vi "Get All Symbol Notifications.vi"(8 "error in (no error)":errorcluster, 11 "TwinCAT ADS in":refnum<class "TwinCAT ADS.lvclass">) -> (0 "error out":errorcluster, 2 "Notification Symbols":T1(array[cluster]), 3 "TwinCAT ADS out":refnum<class "TwinCAT ADS.lvclass">)   [LabVIEW 2018, in "TwinCAT ADS.lvclass"]
uses:
  TwinCAT ADS.lvclass
  TwinCAT ADS.lvclass/TwinCAT ADS.ctl
  Controls/Notifcation Map Value.ctl
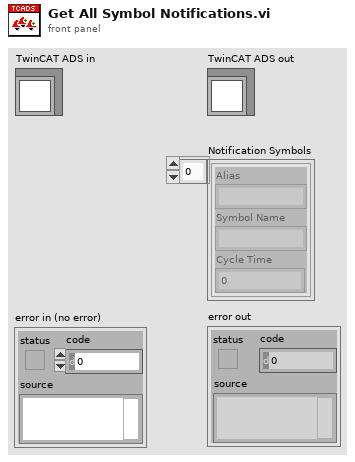
[diagram p1: front panel]
types:
  T1 = cluster{"Alias":string, "Symbol Name":string, "Cycle Time":i32}[]
  T2 = typedef "TwinCAT ADS.lvclass/Notifcation Map Value.ctl" = cluster{"Handle":i32, "Cycle Time":i32}
  T3 = cluster{"Alias":string, "Symbol Name":string, "Cycle Time":i32}
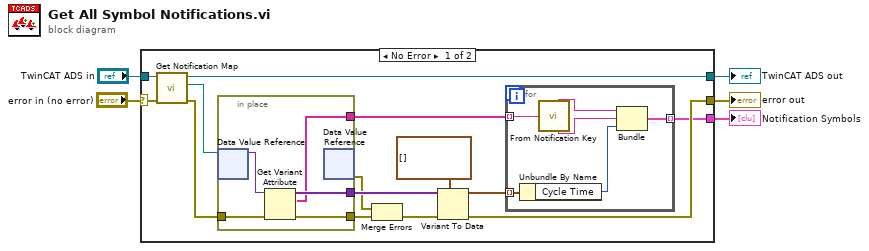
[diagram p0: block diagram]
diagram:
  n1 = case shown="No Error" "error in (no error)" {
    selector: "error in (no error)" -> [w6 w31]
    tunnel: "TwinCAT ADS in" -> [w19 w32]
    tunnel: [w10 w32] -> w4
    tunnel: [w9 w31] -> w2
    tunnel: [w8 _] -> w1
    frame No Error {
      n2 = call "Get Notification Map.vi"("error in (no error)"=w6, "TwinCAT ADS in"=w19) -> ("error out"=w7:errorcluster, "Notification Map"=w18:refnum<data-value>, "TwinCAT ADS out"=w10:refnum<class "TwinCAT ADS.lvclass">)  [unwired: 7 in]
      n3 = in-place {
        in-place-border: [w29] -> w17
        in-place-border: [w28] -> w12
        in-place-border: [w27] -> w16
        in-place-border: w7 -> [w26]
        n4 = in-place-dvr #1(w18) -> (w30:variant)  [unwired: 1 out]
        n5 = Get Variant Attribute(Variant=w30, error in=w26) -> (names=w28:string[], values=w29:variant[], error out=w27:errorcluster)  [unwired: 2 in, 1 out]
        n6 = in-place-dvr #1() -> (w15:errorcluster)  [unwired: 1 in, 1 out]
      }
      n7 = Merge Errors(w15, w16) -> (w14:errorcluster)
      n8 = Variant To Data(error in=w14, type=T2[] [], Variant=w17) -> (data=w11:T2[], error out=w9:errorcluster)
      n9 = for {
        tunnel: w12 -> [w22] mode=indexing
        tunnel: w11 -> [w25] mode=indexing
        tunnel: [w23] -> w8 mode=indexing
        n10 = Unbundle By Name(w25) -> ("Cycle Time"=w24:i32)
        n11 = call "From Notification Key.vi"("Key"=w22) -> ("Alias"=w21:string, "Symbol Name"=w20:string)  [unwired: 7 in]
        n12 = Bundle("Alias"=w21, "Symbol Name"=w20, "Cycle Time"=w24) -> (w23:T3)  [unwired: 1 in]
      }
    }
    frame Error {
    }
  }
  "error out" <- w2
  "TwinCAT ADS out" <- w4
  "Notification Symbols" <- w1
